vi "getClassHierarchy__ogtk.vi"(8 "error in (no error)":errorcluster, 10 "className":string) -> (0 "error out":errorcluster, 2 "classHierarchy":string[](array[string]))   [LabVIEW 2023, in "openg_variant.lvlib" / "Reflection__ogtk.lvclass"]
doc: "Get the class hierarchy for the specified class. The first element of the output array is the top most parent class; the last element is the input class. Input className can include or exclude the '.lvclass' extension. Output values include '.lvclass' extension.\n\nGCraftsman JSON Object Serialization Toolkit\nwww.GCraftsman.com\nCopyright (c) 2017, GCraftsman"
uses:
  Reflection__ogtk.lvclass
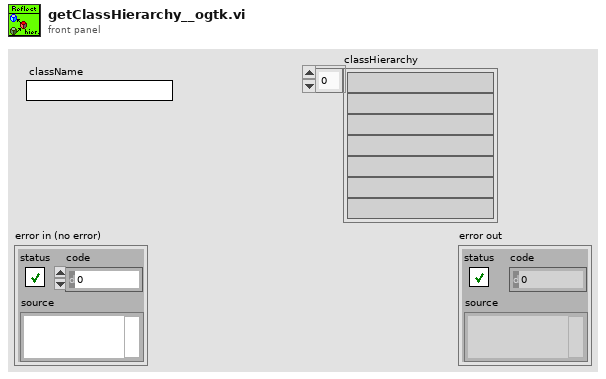
[diagram p1: front panel]
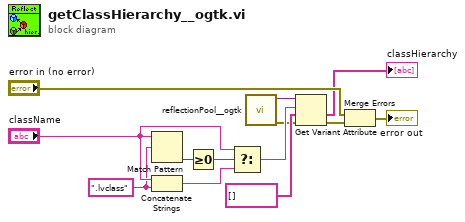
[diagram p0: block diagram]
diagram:
  w8 = ".lvclass" ("regular expression")
  n1 = Match Pattern(string="className", regular expression=w8) -> (offset past match=w11:i32)  [unwired: 1 in, 3 out]
  n2 = Concatenate Strings("className", w8) -> (w7:string)
  n3 = Greater Or Equal To 0?(x=w11) -> (x >= 0?=w10:bool)
  n4 = Select(t="className", s=w10, f=w7) -> (s? t:f=w6:string)
  n5 = call "reflectionPool__ogtk.vi"() -> ("error out"=w1:errorcluster, "classHierarchyLUT"=w5:variant)  [unwired: 6 in, 4 out]
  n6 = Get Variant Attribute(Variant=w5, name=w6, default value (empty Variant)=string[] [] ("classHierarchy"), error in=w1) -> (value=→"classHierarchy":string[], error out=w4:errorcluster)  [unwired: 2 out]
  n7 = Merge Errors("error in (no error)", w4) -> (→"error out":errorcluster)
